vi "piezoWriteUSBOpen.vi"   [LabVIEW 2017]
uses:
  globalDevices.vi
  Piezo/lvlib/Madlib.lvlib
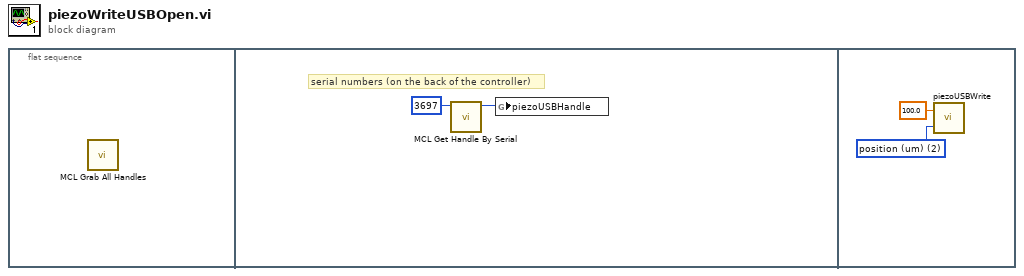
[diagram p0: block diagram]
diagram:
  n1 = flat-sequence {
    frame #0 {
      n2 = call "MCL Grab All Handles.vi"() -> ()  [unwired: 11 in, 1 out]
    }
    frame #1 {
      # "serial numbers (on the back of the controller)"
      n3 = call "MCL Get Handle By Serial.vi"("serial"=i16 3697) -> ("function return"=w1:i32)  [unwired: 10 in]
      n4 = global write "globalDevices.vi" "piezoUSBHandle"(w1) -> ()
    }
    frame #2 {
      w3 = u16 2 items=["fractional", "voltage (V)", "position (um)"] ("mode")
      n5 = call "piezoUSBWrite.vi"("mode"=w3, "position"=100.0) -> ()  [unwired: 1 in]
    }
  }
